vi "Pre Launch Init.vi"(11 "MSS Target Actor in":refnum<class "MSS Target Actor.lvclass">) -> (0 "error out":errorcluster, 3 "MSS Target Actor out":refnum<class "MSS Target Actor.lvclass">)   [LabVIEW 2023, in "MSS Target Actor.lvlib" / "MSS Target Actor.lvclass"]
doc: "(<B>Filename</B>: Actor Framework.lvlib:Actor.lvclass:Pre Launch Init.vi)\n\nDefines behavior that occurs after the Launch Nested Actor method is invoked but before the actor's Actor Core method begins running.\n\nBy default, this method does nothing. A descendant class may override it to define behavior."
uses:
  MSS Target Actor.lvclass
  MSS Target Actor.lvclass/MSS Target Actor.ctl
  <vilib>/ActorFramework/Actor/Actor.lvclass
  Reply-Msg-DataSocket/Reply Msg DataSocket/Reply Msg DataSocket.lvclass
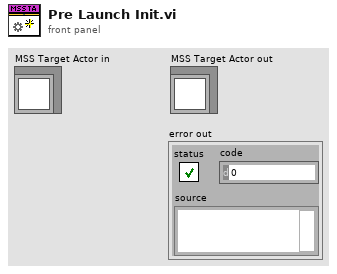
[diagram p1: front panel]
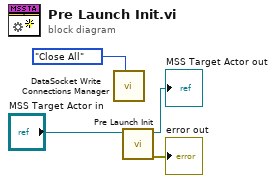
[diagram p0: block diagram]
diagram:
  n1 = call "DataSocket Write Connections Manager.vi"("Action"=enum16{"Get", "Close", "Close All"}."Close All") -> ()  [unwired: 10 in, 1 out]
  n2 = call-parent "Pre Launch Init.vi"("Actor in"="MSS Target Actor in") -> ("error out"=→"error out":errorcluster, "Actor out"=→"MSS Target Actor out":refnum<class "MSS Target Actor.lvclass">)  [unwired: 9 in]
